vi "UpdateErrorList.vi"(0 "tree listbox":refnum<vi>, 5 "error in":errorcluster) -> (19 "error out":errorcluster)   [LabVIEW 2018, in "Error handler.lvclass"]
uses:
  Error handler.lvclass
  <vilib>/Utility/miscctls.llb/LVRowAndColumnTypeDef.ctl
panel:
  # "Missing object. The object \"Map\" does not exist in the previous version."
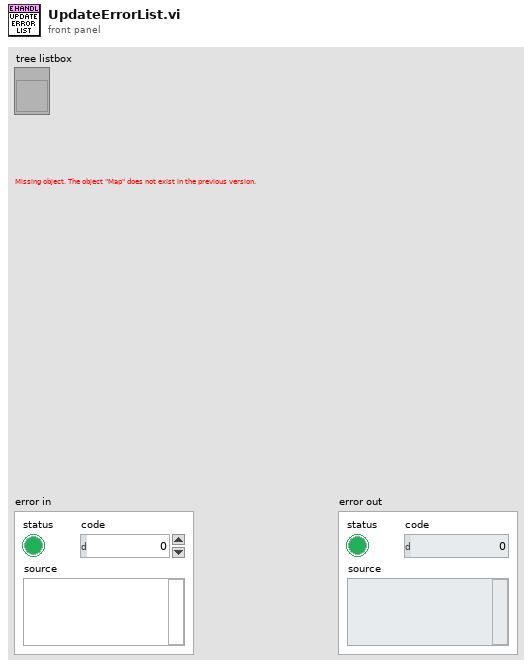
[diagram p1: front panel]
types:
  T1 = typedef "LVRowAndColumnTypeDef.ctl" = cluster{"Row":i32, "Column":i32}
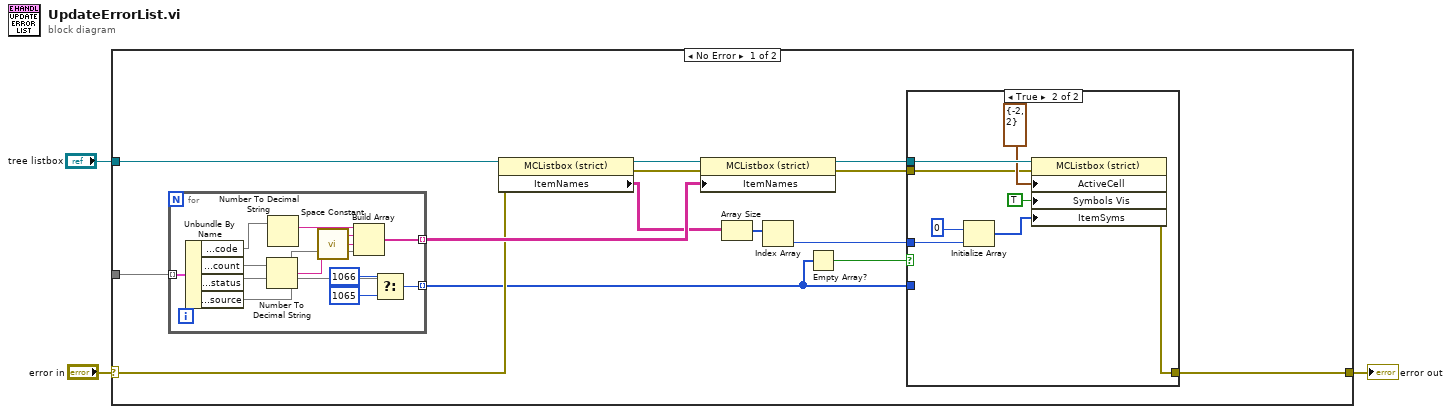
[diagram p0: block diagram]
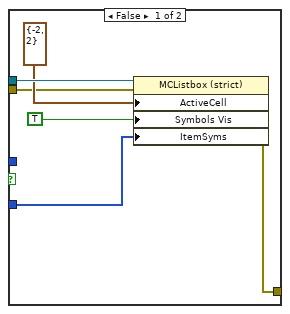
[diagram p2: hidden frame]
diagram:
  n1 = case shown="No Error" "error in" {
    selector: "error in" -> [w10 w44]
    tunnel: [w13 w44] -> w2
    tunnel: "tree listbox" -> [w11 _]
    tunnel: _ -> [w17 _]
    frame No Error {
      n2 = for {
        tunnel: w17 -> [w43] mode=indexing
        tunnel: [w36] -> w16 mode=indexing
        tunnel: [w32] -> w6 mode=indexing
        n3 = Unbundle By Name(w43) -> ("ErrorInformation.error.code"=w42, "ErrorInformation.count"=w41, "ErrorInformation.error.status"=w35, "ErrorInformation.error.source"=w37)
        n4 = Number To Decimal String(number=w41) -> (decimal integer string=w39:string)  [unwired: 1 in]
        n5 = Number To Decimal String(number=w42) -> (decimal integer string=w40:string)  [unwired: 1 in]
        n6 = call <vilib>:"Space Constant.vi"() -> ("String"=w38:string)
        n7 = Build Array(w40, w39, w38, w37) -> (w36:string[])
        n8 = Select(t=1066, s=w35, f=1065) -> (s? t:f=w32:i32)
      }
      n9 = property class="MCListbox (strict)"(reference=w11, error in=w10) -> (reference out=w12:refnum<vi>, error out=w9:errorcluster, "ItemNames"=w8:string[][])
      n10 = property class="MCListbox (strict)"(reference=w12, error in=w9, "ItemNames"=w16) -> (reference out=w15:refnum<vi>, error out=w14:errorcluster)
      n11 = Array Size(array=w8) -> (size(s)=w7:i32[])
      n12 = Index Array(array=w7) -> (element=w4:i32)  [unwired: 1 in]
      n13 = Empty Array?(array=w6) -> (empty?=w5:bool)
      n14 = case shown="True" w5 {
        tunnel: w15 -> [w23 w31]
        tunnel: w14 -> [w20 w28]
        tunnel: [w19 w27] -> w13
        tunnel: w6 -> [w18 _]
        tunnel: w4 -> [_ w26]
        frame False {
          n15 = property class="MCListbox (strict)"(reference=w23, error in=w20, "ActiveCell"=T1 {"Row"=-2, "Column"=2} ("Active Cell:Active Cell"), "Symbols Vis"=TRUE ("Visible Items:Symbols Visible"), "ItemSyms"=w18) -> (error out=w19:errorcluster)  [unwired: 1 out]
        }
        frame True {
          n16 = Initialize Array(0, w26) -> (w24:i32[])
          n17 = property class="MCListbox (strict)"(reference=w31, error in=w28, "ActiveCell"=T1 {"Row"=-2, "Column"=2} ("Active Cell:Active Cell"), "Symbols Vis"=TRUE ("Visible Items:Symbols Visible"), "ItemSyms"=w24) -> (error out=w27:errorcluster)  [unwired: 1 out]
        }
      }
    }
    frame Error {
    }
  }
  "error out" <- w2
